vi "Sine Generator (Host).vi"() -> ()   [LabVIEW 2012]
doc: "This host VI converts real-world signal parameters from floating-point units of Hz, degrees, and volts to scaled fixed-point units appropriate for FPGA execution."
uses:
  <vilib>/rvi/interface/nirviReadWriteControl/nirviReadWriteControl.xnode
  <vilib>/rvi/interface/nirviCloseFPGA/nirviCloseFPGA.xnode
  <vilib>/rvi/interface/nirviOpenFPGA/nirviOpenFPGA.xnode
  <vilib>/rvi/Analysis/host/Public/NI_FpgaMspHost.lvlib
  <vilib>/rvi/Analysis/host/Private/Sample Rate To Loop Time (ticks).vi
  Sine Generator (FPGA).vi
  NiFpgaLv.dll
  <vilib>/Utility/error.llb/Error Cluster From Error Code.vi
  <vilib>/rvi/errors/niLvFpgaAdjustHostInterfaceError.vi
  <vilib>/FPGAPlugInAG/PXI-7831R/niLvFpga_Close_PXI-7831R.vi
panel:
  in  "Reset":bool
  out "Nyquist warning 1":bool
  in  "Sine wave 1":T1={"Sine wave frequency (Hz)"=2000.0, "Phase offset (deg)"=180.0, "Vpeak (V)"=6.0, "Voffset (V)"=0.0} {"Phase offset (deg)" format="%#_6p"; "Sine wave frequency (Hz)" format="%#_6p"}
  in  "Sine wave 0":T1={"Sine wave frequency (Hz)"=1000.0, "Phase offset (deg)"=0.0, "Vpeak (V)"=10.0, "Voffset (V)"=0.0} {"Phase offset (deg)" format="%#_6p"; "Sine wave frequency (Hz)" format="%#_6p"}
  in  "Sample rate (S/s)":dbl=400000.0 format="%#_6p"
  out "Nyquist warning 0":bool
  out "Actual sample rate (S/s)":dbl=100000.0 format="%#_6p"
  out "Sampling rate achieved?":bool=TRUE
  in  "Stop":bool
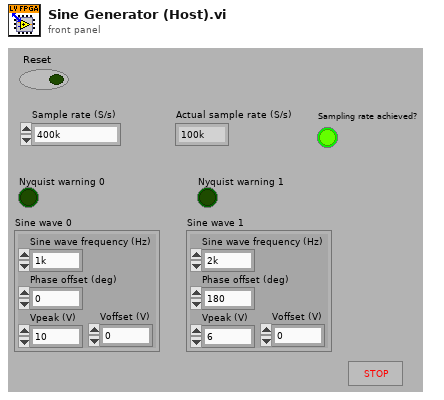
[diagram p1: front panel]
types:
  T1 = cluster{"Sine wave frequency (Hz)":dbl, "Phase offset (deg)":dbl, "Vpeak (V)":dbl, "Voffset (V)":dbl}
  T2 = cluster{"Frequency (periods/tick)":fxp<+,32,0>, "Phase offset (periods)":fxp<+,32,0>, "Scale factor":fxp<+/-,16,1>, "Amplitude offset":fxp<+/-,16,16>}
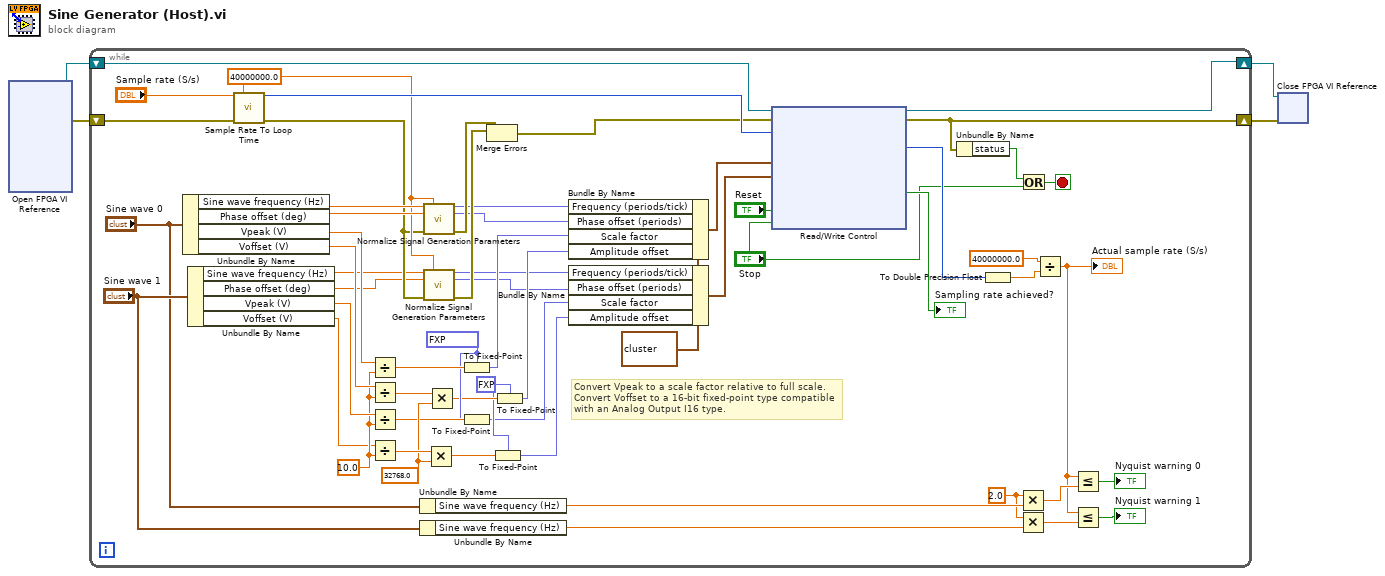
[diagram p0: block diagram]
diagram:
  n1 = xnode "Open FPGA VI Reference"() -> ("FPGA VI Reference Out"=w4:refnum<k20>, "error out"=w3:errorcluster)  [unwired: 2 in]
  n2 = while {
    shift-right: [w50] -> w2
    shift-left: w3 -> [w45]
    shift-right: [w33] -> w1
    shift-left: w4 -> [w62]
    stop <- w48 stop-if-true
    w18 = fxp<+/-,16,16> 0.0 ("Amplitude offset")
    w20 = fxp<+/-,16,1> 0.999969482421875 ("Scale factor")
    w23 = 32768.0 ("y")
    w29 = 10.0 ("y")
    w8 = T2 {"Frequency (periods/tick)"=0.0, "Phase offset (periods)"=0.0, "Scale factor"=0.999969482421875, "Amplitude offset"=0.0} ("Sinewave Props 0")
    w5 = 2.0 ("x")
    w40 = 40000000.0 ("x")
    # "Convert Vpeak to a scale factor relative to full scale.\nConvert Voffset to a 16-bit fixed-point type compatible \nwith an Analog Output I16 type."
    n3 = Unbundle By Name("Sine wave 0") -> ("Sine wave frequency (Hz)"=w42:dbl, "Phase offset (deg)"=w41:dbl, "Vpeak (V)"=w32:dbl, "Voffset (V)"=w30:dbl)
    n4 = Unbundle By Name("Sine wave 1") -> ("Sine wave frequency (Hz)"=w27:dbl, "Phase offset (deg)"=w26:dbl, "Vpeak (V)"=w31:dbl, "Voffset (V)"=w28:dbl)
    n5 = call-poly <vilib>:"Sample Rate To Loop Time.vi"("sample rate (S/s)"="Sample rate (S/s)", "FPGA clock rate (Hz)"=w40, "error in (no error)"=w45) -> ("count (ticks/S)"=w43:u32, "error out"=w37:errorcluster)  [unwired: 10 in, 1 out]
    n6 = Divide(x=w32, y=w29) -> (x/y=w22:dbl)
    n7 = Divide(x=w30, y=w29) -> (x/y=w25:dbl)
    n8 = Divide(x=w31, y=w29) -> (x/y=w21:dbl)
    n9 = Divide(x=w28, y=w29) -> (x/y=w24:dbl)
    n10 = Unbundle By Name("Sine wave 0") -> ("Sine wave frequency (Hz)"=w38:dbl)
    n11 = Unbundle By Name("Sine wave 1") -> ("Sine wave frequency (Hz)"=w53:dbl)
    n12 = call <vilib>:"Normalize Signal Generation Parameters.vi"("frequency (Hz)"=w42, "FPGA clock rate (Hz)"=w40, "phase offset (deg)"=w41, "error in (no error)"=w37) -> ("frequency (periods/tick)"=w16:fxp<+,32,0>, "phase offset (periods)"=w15:fxp<+,32,0>, "error out"=w36:errorcluster)  [unwired: 6 in, 3 out]
    n13 = call <vilib>:"Normalize Signal Generation Parameters.vi"("frequency (Hz)"=w27, "FPGA clock rate (Hz)"=w40, "phase offset (deg)"=w26, "error in (no error)"=w37) -> ("frequency (periods/tick)"=w12:fxp<+,32,0>, "phase offset (periods)"=w11:fxp<+,32,0>, "error out"=w35:errorcluster)  [unwired: 6 in, 3 out]
    n14 = Multiply(x=w24, y=w23) -> (x*y=w17:dbl)
    n15 = Multiply(x=w25, y=w23) -> (x*y=w19:dbl)
    n16 = To Fixed-Point(fixed-point type=w20, number=w22) -> (fixed-point=w14:fxp<+/-,16,1>)
    n17 = To Fixed-Point(fixed-point type=w20, number=w21) -> (fixed-point=w10:fxp<+/-,16,1>)
    n18 = Merge Errors(w36, w35) -> (w34:errorcluster)
    n19 = To Fixed-Point(fixed-point type=w18, number=w17) -> (fixed-point=w9:fxp<+/-,16,16>)
    n20 = To Fixed-Point(fixed-point type=w18, number=w19) -> (fixed-point=w13:fxp<+/-,16,16>)
    n21 = Bundle By Name(cluster=w8, "Frequency (periods/tick)"=w16, "Phase offset (periods)"=w15, "Scale factor"=w14, "Amplitude offset"=w13) -> (w7:T2)
    n22 = Bundle By Name(cluster=w8, "Frequency (periods/tick)"=w12, "Phase offset (periods)"=w11, "Scale factor"=w10, "Amplitude offset"=w9) -> (w6:T2)
    n23 = xnode "Read/Write Control"("FPGA VI Reference In"=w62, "error in"=w34, "Desired loop rate (ticks)"=w43, "Sinewave Props 0"=w7, "Sinewave Props 1"=w6, "Initialize"="Reset", "Stop"="Stop") -> ("FPGA VI Reference Out"=w33:refnum<k20>, "error out"=w50:errorcluster, "Actual loop rate"=w60:u32, "Sampling rate achieved?"=→"Sampling rate achieved?":bool)
    n24 = Unbundle By Name(w50) -> ("status"=w49:bool)
    n25 = To Double Precision Float(number=w60) -> (double precision float=w59:dbl)
    n26 = Multiply(x=w5, y=w38) -> (x*y=w57:dbl)
    n27 = Multiply(x=w5, y=w53) -> (x*y=w54:dbl)
    n28 = Or(x=w49, y="Stop") -> (x .or. y?=w48:bool)
    n29 = Divide(x=40000000.0 ("y"), y=w59) -> (x/y=w52:dbl)
    "Actual sample rate (S/s)" <- w52
    n30 = Less Or Equal?(x=w52, y=w57) -> (x <= y?=→"Nyquist warning 0":bool)
    n31 = Less Or Equal?(x=w52, y=w54) -> (x <= y?=→"Nyquist warning 1":bool)
  }
  n32 = xnode "Close FPGA VI Reference"("FPGA VI Reference In"=w1, "error in"=w2) -> ()  [unwired: 1 out]
